vi "_Load Config File.vi"(2 "error in (no error)":errorcluster) -> (0 "error out":errorcluster, 1 "Instrument":string[](array[string]))   [LabVIEW 2018]
uses:
  Type/_RT Command.ctl
  Type/_RT Configuration 2.ctl
  Configuration/_Global Configuration.vi
  <vilib>/Utility/config.llb/Read Key (I32).vi
  <vilib>/Utility/config.llb/Read Key (Boolean).vi
  <vilib>/Utility/config.llb/Read Key (String).vi
  <vilib>/Utility/config.llb/Write Key (String).vi
  <vilib>/Utility/config.llb/NI_LVConfig.lvlib
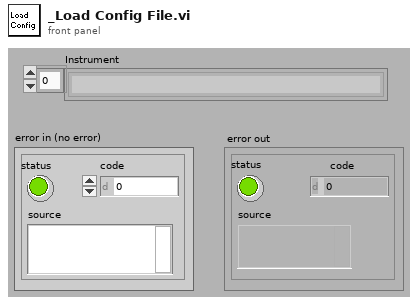
[diagram p1: front panel]
types:
  T1 = typedef "_RT Command.ctl" = enum16{"xml Start Run", "xml Start Actual Run", "xml Stop Run", "xml Runtime Update", "xml Get Status", "xml Get Table", "xml Set Table", "xml Get Configuration", "xml System Status", "xml Set LC Input Logic", "xml Get Data", "xml Get Info", "Start", "StartActualRun", "Stop", "Runtime Update", "Get Data", "Get Info", "Get Status", "Get Param", "Get Config", "Get Table", "Read ADC", "Set Oscillator", "Update Config", "Update Table", "Set All Pol", "Set Pol and DC", "Set Max Mass", "Toggle RP", "Toggle EL", "Set PIC", "Initialize Turbo", "Send Turbo Comm", "Close Turbo", "P1", "P2", "P3", "Send Serial", "Set LC Out", "Get LC In", "Read VAC", "Test Table", "Toggle Power", "Get Startup", "Set Startup", "Get ADC Table", "Set ADC Table", "Get Brief Status", "Get Detail Status", "Auxiliary Update", "Set CC Logics", "Set CC Input Logics", "Ignore Error", "invalid"}
  T2 = typedef "NI_LVConfig.lvlib/Config Data RefNum.ctl" = refnum<k1>
  T3 = typedef "_RT Instrument 2.ctl" = cluster{"Table":T4[], "Instrument":string[]}
  T4 = typedef "_RT Configuration 2.ctl" = cluster{"Name":string, "Ch#":u8, "Min":dbl, "Max":dbl, "Def+":dbl, "Def-":dbl, "Offset":dbl, "Slope":dbl, "Type":u8, "Description":string, "SettleT":dbl}
  T5 = typedef "_Instrument Model.ctl" = enum16{"QSight 110", "QSight 120", "QSight 210", "QSight 220", "QSight 410", "QSight 420", "IONICS 3Q 110", "IONICS 3Q 120", "IONICS 3Q 210", "IONICS 3Q 220", "IONICS 3Q 310", "IONICS 3Q 320", "Simulation (Single Source)", "Simulation (Dual Source)"}
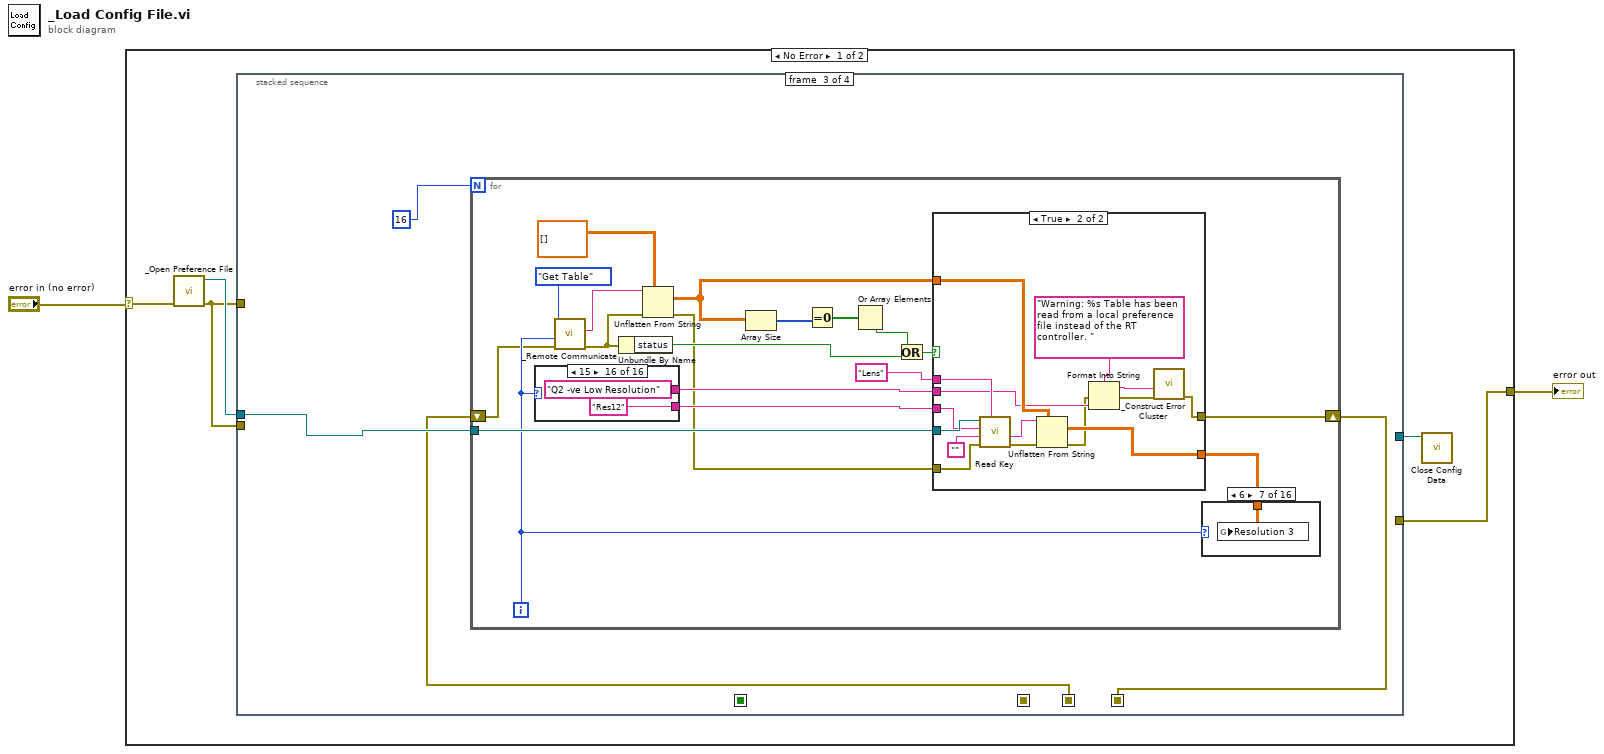
[diagram p0: block diagram]
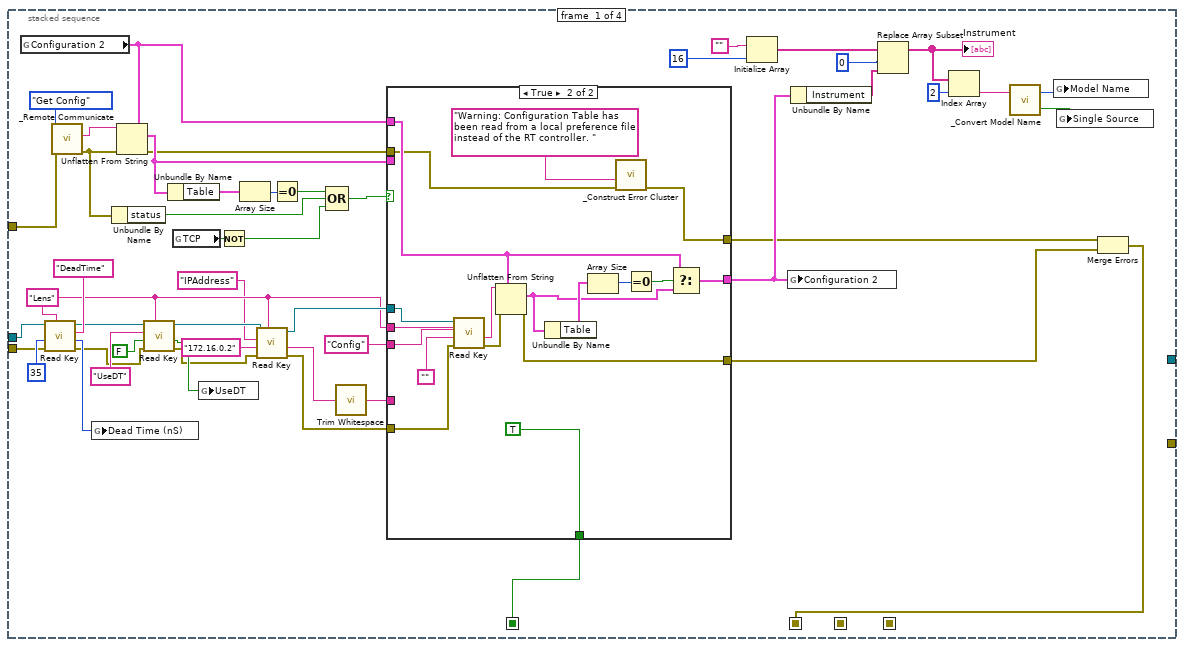
[diagram p2: hidden frame]
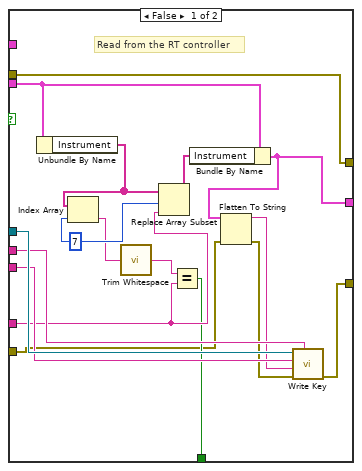
[diagram p3: hidden frame]
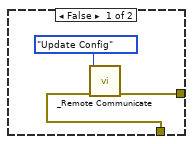
[diagram p5: hidden frame]
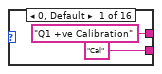
[diagram p6: hidden frame]
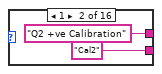
[diagram p7: hidden frame]
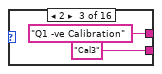
[diagram p8: hidden frame]
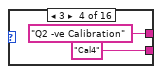
[diagram p9: hidden frame]
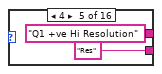
[diagram p10: hidden frame]
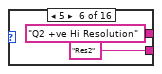
[diagram p11: hidden frame]
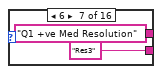
[diagram p12: hidden frame]
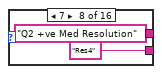
[diagram p13: hidden frame]
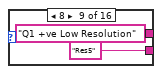
[diagram p14: hidden frame]
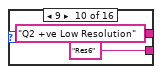
[diagram p15: hidden frame]
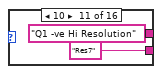
[diagram p16: hidden frame]
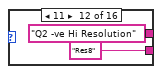
[diagram p17: hidden frame]
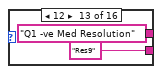
[diagram p18: hidden frame]
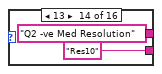
[diagram p19: hidden frame]
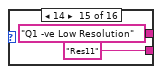
[diagram p20: hidden frame]
diagram:
  n1 = case shown="No Error" "error in (no error)" {
    selector: "error in (no error)" -> [w5 w241]
    tunnel: [w3 w241] -> w1
    frame No Error {
      n2 = call "_Open Preference File.vi"("error In"=w5) -> ("error"=w4:errorcluster, "refnum"=w7:T2)  [unwired: 2 in, 3 out]
      n3 = stacked-sequence {
        seq-local: [w21 _ _ _] -> [_ w94 _ _]
        seq-local: [w8 _ _ _] -> [_ w93 _ _]
        seq-local: [_ w92 _ _] -> [_ _ w100 _]
        seq-local: [_ _ w99 _] -> [_ _ _ w196]
        tunnel: w7 -> [w31 _ w101 w198]
        tunnel: [_ _ _ w197] -> w6
        tunnel: w4 -> [w17 _ _ _]
        tunnel: w4 -> [w15 _ _ _]
        tunnel: [_ _ _ w193] -> w3
        frame #0 {
          w26 = "Lens" ("section")
          n4 = global read "_Global Configuration.vi" "Configuration 2"() -> (w36:T3)
          n5 = call-poly <vilib>:"Read Key.vi"("section"=w26, "error in (no error)"=w15, "default value"=35, "key"="DeadTime", "refnum"=w31) -> ("error out"=w14:errorcluster, "value"=w50:i32, "refnum out"=w49:T2)  [unwired: 4 out]
          n6 = call "_Remote Communicate.vi"("error in (no error)"=w17, "Command"=_RT_Command."Get Config") -> ("error out"=w16:errorcluster, "Info"=w52:string)  [unwired: 4 in, 2 out]
          n7 = global write "_Global Configuration.vi" "Dead Time (nS)"(w50) -> ()
          n8 = Unbundle By Name(w16) -> ("status"=w55:bool)
          n9 = Unflatten From String(type=w36, binary string=w52, error in (no error)=w16) -> (value=w33:T3, error out=w11:errorcluster)  [unwired: 3 out]
          n10 = call-poly <vilib>:"Read Key.vi"("section"=w26, "error in (no error)"=w14, "default value"=FALSE, "key"="UseDT", "refnum"=w49) -> ("error out"=w13:errorcluster, "value"=w45:bool, "refnum out"=w28:T2)  [unwired: 4 out]
          n11 = Unbundle By Name(w33) -> ("Table"=w35:T4[])
          n12 = global read "_Global Configuration.vi" "TCP"() -> (w30:bool)
          n13 = global write "_Global Configuration.vi" "UseDT"(w45) -> ()
          n14 = Not(x=w30) -> (.not. x?=w29:bool)
          n15 = Array Size(array=w35) -> (size(s)=w34:i32)
          n16 = call-poly <vilib>:"Read Key.vi"("section"=w26, "error in (no error)"=w13, "default value"="172.16.0.2", "key"="IPAddress" ("section"), "refnum"=w28) -> ("error out"=w12:errorcluster, "value"=w23:string, "refnum out"=w27:T2)  [unwired: 1 in, 3 out]
          n17 = Equal To 0?(x=w34) -> (x = 0?=w32:bool)
          n18 = Compound Arithmetic op=OR(w32, w55, w29) -> (w54:bool)
          n19 = call <vilib>:"Trim Whitespace.vi"("string"=w23) -> ("trimmed string"=w22:string)  [unwired: 1 in]
          n20 = case shown="True" w54 {
            tunnel: w33 -> [w70 _]
            tunnel: [w61 w79] -> w43
            tunnel: w27 -> [w73 w91]
            tunnel: w26 -> [w72 w88]
            tunnel: "Config" ("section") -> [w71 w86]
            tunnel: [w57 w87] -> w9
            tunnel: w36 -> [_ w80]
            tunnel: w22 -> [w63 _]
            tunnel: [w62 TRUE] -> w21
            tunnel: w12 -> [w60 w77]
            tunnel: w11 -> [w57 w74]
            tunnel: [w58 w75] -> w10
            frame False {
              w66 = 7 ("index")
              # "Read from the RT controller"
              n21 = Unbundle By Name(w70) -> ("Instrument"=w67:string[])
              n22 = Index Array(array=w67, index=w66) -> (element=w65:string)
              n23 = call <vilib>:"Trim Whitespace.vi"("string"=w65) -> ("trimmed string"=w64:string)  [unwired: 1 in]
              n24 = Replace Array Subset(array=w67, new element=w63, index=w66) -> (w69:string[])
              n25 = Equal?(x=w64, y=w63) -> (x = y?=w62:bool)
              n26 = Bundle By Name(cluster=w70, "Instrument"=w69) -> (w61:T3)
              n27 = Flatten To String(anything=w61, error in (no error)=w60) -> (data string=w68:string, error out=w59:errorcluster)  [unwired: 3 out]
              n28 = call-poly <vilib>:"Write Key.vi"("section"=w72, "error in (no error)"=w59, "value"=w68, "key"=w71, "refnum"=w73) -> ("error out"=w58:errorcluster)  [unwired: 1 in, 5 out]
            }
            frame True {
              n29 = call-poly <vilib>:"Read Key.vi"("section"=w88, "error in (no error)"=w77, "default value"="", "key"=w86, "refnum"=w91) -> ("error out"=w76:errorcluster, "value"=w89:string)  [unwired: 1 in, 4 out]
              n30 = Unflatten From String(type=w80, binary string=w89, error in (no error)=w76) -> (value=w81:T3, error out=w75:errorcluster)  [unwired: 3 out]
              n31 = Unbundle By Name(w81) -> ("Table"=w83:T4[])
              n32 = Array Size(array=w83) -> (size(s)=w84:i32)
              n33 = call "_Construct Error Cluster.vi"("error in"=w74, "reason"="Warning: Configuration Table has been read from a local preference file instead of the RT controller. ") -> ("error out"=w87:errorcluster)  [unwired: 2 in, 3 out]
              n34 = Equal To 0?(x=w84) -> (x = 0?=w82:bool)
              n35 = Select(t=w80, s=w82, f=w81) -> (s? t:f=w79:T3)
            }
          }
          n36 = Initialize Array("", 16 ("dimension size")) -> (w40:string[])
          n37 = global write "_Global Configuration.vi" "Configuration 2"(w43) -> ()
          n38 = Unbundle By Name(w43) -> ("Instrument"=w38:string[])
          n39 = Replace Array Subset(array=w40, new element=w38, index=0) -> (w37:string[])
          "Instrument" <- w37
          n40 = Index Array(array=w37, index=2) -> (element=w20:string)
          n41 = call "_Convert Model Name.vi"("Model"=w20) -> ("SingleSource"=w19:bool, "Model Name"=w18:T5)  [unwired: 1 in]
          n42 = global write "_Global Configuration.vi" "Model Name"(w18) -> ()
          n43 = global write "_Global Configuration.vi" "Single Source"(w19) -> ()
          n44 = Merge Errors(w9, w10) -> (w8:errorcluster)
        }
        frame #1 {
          n45 = case shown="True" w94 {
            tunnel: [w96 w98] -> w92
            tunnel: w93 -> [w95 w98]
            frame False {
              n46 = call "_Remote Communicate.vi"("error in (no error)"=w95, "Command"=_RT_Command."Update Config") -> ("error out"=w96:errorcluster)  [unwired: 4 in, 3 out]
            }
            frame True {
            }
          }
        }
        frame #2 {
          n47 = for {
            N: 16 -> [_]
            tunnel: w101 -> [w120]
            shift-right: [w103] -> w99
            shift-left: w100 -> [w106]
            i -> [w109]
            n48 = case shown="15" w109 {
              tunnel: ["Q1 +ve Calibration" ("section") "Q2 +ve Calibration" ("section") "Q1 -ve Calibration" ("section") "Q2 -ve Calibration" ("section") "Q1 +ve Hi Resolution" ("section") "Q2 +ve Hi Resolution" ("section") "Q1 +ve Med Resolution" ("section") "Q2 +ve Med Resolution" ("section") "Q1 +ve Low Resolution" ("section") "Q2 +ve Low Resolution" ("section") "Q1 -ve Hi Resolution" ("section") "Q2 -ve Hi Resolution" ("section") "Q1 -ve Med Resolution" ("section") "Q2 -ve Med Resolution" ("section") "Q1 -ve Low Resolution" ("section") "Q2 -ve Low Resolution" ("section")] -> w107
              tunnel: ["Cal" ("section") "Cal2" ("section") "Cal3" ("section") "Cal4" ("section") "Res" ("section") "Res2" ("section") "Res3" ("section") "Res4" ("section") "Res5" ("section") "Res6" ("section") "Res7" ("section") "Res8" ("section") "Res9" ("section") "Res10" ("section") "Res11" ("section") "Res12" ("section")] -> w108
              frame 0, Default {
              }
              frame 1 {
              }
              frame 2 {
              }
              frame 3 {
              }
              frame 4 {
              }
              frame 5 {
              }
              frame 6 {
              }
              frame 7 {
              }
              frame 8 {
              }
              frame 9 {
              }
              frame 10 {
              }
              frame 11 {
              }
              frame 12 {
              }
              frame 13 {
              }
              frame 14 {
              }
              frame 15 {
              }
            }
            n49 = call "_Remote Communicate.vi"("error in (no error)"=w106, "DC Param"=w109, "Command"=_RT_Command."Get Table") -> ("error out"=w105:errorcluster, "Info"=w119:string)  [unwired: 3 in, 2 out]
            n50 = Unbundle By Name(w105) -> ("status"=w117:bool)
            n51 = Unflatten From String(type=dbl[][] [] ("Cal-"), binary string=w119, error in (no error)=w105) -> (value=w111:dbl[][], error out=w104:errorcluster)  [unwired: 3 out]
            n52 = Array Size(array=w111) -> (size(s)=w114:i32[])
            n53 = Equal To 0?(x=w114) -> (x = 0?=w113:bool[])
            n54 = Or Array Elements(Boolean array=w113) -> (logical OR=w112:bool)
            n55 = Or(x=w112, y=w117) -> (x .or. y?=w116:bool)
            n56 = case shown="True" w116 {
              tunnel: [w174 w190] -> w110
              tunnel: w120 -> [w177 w192]
              tunnel: "Lens" ("section") -> [w176 w188]
              tunnel: w108 -> [w175 w186]
              tunnel: [w170 w187] -> w103
              tunnel: w111 -> [w174 w185]
              tunnel: w107 -> [_ w184]
              tunnel: w104 -> [w172 w180]
              frame False {
                # "Read from the RT controller"
                n57 = Flatten To String(anything=w174, error in (no error)=w172) -> (data string=w173:string, error out=w171:errorcluster)  [unwired: 3 out]
                n58 = call-poly <vilib>:"Write Key.vi"("section"=w176, "error in (no error)"=w171, "value"=w173, "key"=w175, "refnum"=w177) -> ("error out"=w170:errorcluster)  [unwired: 1 in, 5 out]
              }
              frame True {
                n59 = call-poly <vilib>:"Read Key.vi"("section"=w188, "error in (no error)"=w180, "default value"="", "key"=w186, "refnum"=w192) -> ("error out"=w179:errorcluster, "value"=w189:string)  [unwired: 1 in, 4 out]
                n60 = Unflatten From String(type=w185, binary string=w189, error in (no error)=w179) -> (value=w190:dbl[][], error out=w178:errorcluster)  [unwired: 3 out]
                n61 = Format Into String(format string="Warning: %s Table has been read from a local preference file instead of the RT controller. ", error in=w178, w184) -> (resulting string=w182:string, error out=w181:errorcluster)  [unwired: 1 in]
                n62 = call "_Construct Error Cluster.vi"("error in"=w181, "reason"=w182) -> ("error out"=w187:errorcluster)  [unwired: 2 in, 3 out]
              }
            }
            n63 = case shown="6" w109 {
              tunnel: w110 -> [w154 w155 w156 w157 w158 w159 w160 w161 w162 w163 w164 w165 w166 w167 w168 w169]
              frame 0, Default {
                n64 = global write "_Global Configuration.vi" "Calibration"(w154) -> ()
              }
              frame 1 {
                n65 = global write "_Global Configuration.vi" "Calibration 2"(w155) -> ()
              }
              frame 2 {
                n66 = global write "_Global Configuration.vi" "Calibration 3"(w156) -> ()
              }
              frame 3 {
                n67 = global write "_Global Configuration.vi" "Calibration 4"(w157) -> ()
              }
              frame 4 {
                n68 = global write "_Global Configuration.vi" "Resolution"(w158) -> ()
              }
              frame 5 {
                n69 = global write "_Global Configuration.vi" "Resolution 2"(w159) -> ()
              }
              frame 6 {
                n70 = global write "_Global Configuration.vi" "Resolution 3"(w160) -> ()
              }
              frame 7 {
                n71 = global write "_Global Configuration.vi" "Resolution 4"(w161) -> ()
              }
              frame 8 {
                n72 = global write "_Global Configuration.vi" "Resolution 5"(w162) -> ()
              }
              frame 9 {
                n73 = global write "_Global Configuration.vi" "Resolution 6"(w163) -> ()
              }
              frame 10 {
                n74 = global write "_Global Configuration.vi" "Resolution 7"(w164) -> ()
              }
              frame 11 {
                n75 = global write "_Global Configuration.vi" "Resolution 8"(w165) -> ()
              }
              frame 12 {
                n76 = global write "_Global Configuration.vi" "Resolution 9"(w166) -> ()
              }
              frame 13 {
                n77 = global write "_Global Configuration.vi" "Resolution 10"(w167) -> ()
              }
              frame 14 {
                n78 = global write "_Global Configuration.vi" "Resolution 11"(w168) -> ()
              }
              frame 15 {
                n79 = global write "_Global Configuration.vi" "Resolution 12"(w169) -> ()
              }
            }
          }
        }
        frame #3 {
          w202 = T4[] []  # ADC Table
          n80 = call "_Remote Communicate.vi"("error in (no error)"=w196, "Command"=_RT_Command."Get ADC Table") -> ("error out"=w195:errorcluster, "Info"=w203:string)  [unwired: 4 in, 2 out]
          n81 = Unflatten From String(type=w202, binary string=w203, error in (no error)=w195) -> (value=w199:T4[], error out=w194:errorcluster)  [unwired: 3 out]
          n82 = Array Size(array=w199) -> (size(s)=w201:i32)
          n83 = Greater Than 0?(x=w201) -> (x > 0?=w200:bool)
          n84 = case shown="True" w200 {
            tunnel: w199 -> [_ w211]
            tunnel: w198 -> [w206 w210]
            tunnel: [w206 w209] -> w197
            tunnel: w194 -> [w205 w208]
            tunnel: [w205 w207] -> w193
            frame False {
            }
            frame True {
              n85 = for {
                tunnel: w211 -> [w230] mode=indexing
                tunnel: w210 -> [w217]
                tunnel: [w214] -> w209
                tunnel: w208 -> [w213]
                tunnel: [w212] -> w207
                i -> [w216]
                w220 = "0"
                w225 = i16 3 ("precision (6)")
                n86 = Unbundle By Name(w230) -> ("Name"=w223:string, "Offset"=w229:dbl, "Slope"=w228:dbl, "Min"=w227:dbl, "Max"=w226:dbl)
                n87 = Number To Fractional String(number=w229) -> (F-format string=w222:string)  [unwired: 3 out]
                n88 = Number To Decimal String(number=w216) -> (decimal integer string=w224:string)  [unwired: 1 out]
                n89 = Number To Fractional String(number=w228) -> (F-format string=w221:string)  [unwired: 3 out]
                n90 = Number To Fractional String(number=w227, precision (6)=w225) -> (F-format string=w219:string)  [unwired: 2 out]
                n91 = Number To Fractional String(number=w226, precision (6)=w225) -> (F-format string=w218:string)  [unwired: 2 out]
                n92 = Build Array(w224, w223, w220, w222, w221, w220, w219, w218) -> (w215:string[])
                n93 = for {
                  tunnel: w217 -> [w240]
                  tunnel: w216 -> [w238]
                  tunnel: w215 -> [w234] mode=indexing
                  tunnel: [w233] -> w214
                  tunnel: w213 -> [w232]
                  tunnel: [w231] -> w212
                  i -> [w239]
                  n94 = Format Into String(format string="Row%d-Col%d" ("section"), w238, w239) -> (resulting string=w236:string)  [unwired: 2 in, 1 out]
                  n95 = call-poly <vilib>:"Write Key.vi"("section"="ADC", "error in (no error)"=w232, "value"=w234, "key"=w236, "refnum"=w240) -> ("error out"=w231:errorcluster, "refnum out"=w233:T2)  [unwired: 1 in, 4 out]
                }
              }
            }
          }
        }
      }
      n96 = call <vilib>:"Close Config Data.vi"("refnum"=w6) -> ()  [unwired: 2 in, 9 out]
    }
    frame Error {
    }
  }
  "error out" <- w1
